vi "PH_GUI.Sevencolor.vi"(1 "State":i32 caption="index") -> (0 "Color Box":u32(colorbox))   [LabVIEW 2014, in "PH_Common.lvlib"]
doc: "By this VI seven colors of a color box are defined by the \"State\":\n\n0 -> blue (suggested meaning: no information available)\n1 -> darkgreen (suggested meaning: stand by/off)\n2 -> lightgreen (suggested meaning: on)\n3 -> yellow (suggested meaning: warning)\n4 -> red (suggested meaning: alarm/malfunction)\n5 -> black (suggested meaning: not implemented)\n6 -> light grey (suggestetd meaning: further meaning)"
uses:
  PH_Common.lvlib
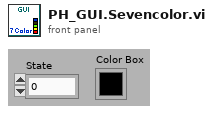
[diagram p1: front panel]
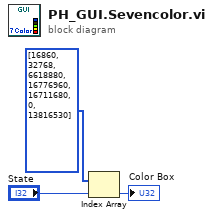
[diagram p0: block diagram]
diagram:
  n1 = Index Array(array=u32[] [16860, 32768, 6618880, 16776960, 16711680, 0, 13816530], index="State") -> (element=→"Color Box":u32)
